vi "bats.parser.common.vi"(11 "BATS.Parser.State.Data in":T1={"BATS.Parser.States"=enum."Send.Command", "Saved.BATS.Parser.State"=enum."Reset", "Hdr Length (U16)"=0, "MessageLength (U8)"=0, "MessageType (U8)"=0, "Time (U32)"=0, "Total Counter (U16)"=0, "Message Counter (U8)"=0, "i"=0, "Number.of.Tickers"=0, "n"=0, "msg.counter"=0, "msg.length"=0, "buffer.start"=0, "buffer.length"=0, "buffer"=[0, 0, 0, 0, 0, 0, 0, 0, 0], "Debug"={"Write.to.Debug"=FALSE, "Data"=0}}) -> (1 "MessageType (U8)":u8, 2 "Message Counter (U8)":u8, 3 "BATS.Parser.State.Data out":T1={"BATS.Parser.States"=enum."Send.Command", "Saved.BATS.Parser.State"=enum."Reset", "Hdr Length (U16)"=0, "MessageLength (U8)"=0, "MessageType (U8)"=0, "Time (U32)"=0, "Total Counter (U16)"=0, "Message Counter (U8)"=0, "i"=0, "Number.of.Tickers"=0, "n"=0, "msg.counter"=0, "msg.length"=0, "buffer.start"=0, "buffer.length"=0, "buffer"=[0, 0, 0, 0, 0, 0, 0, 0, 0], "Debug"={"Write.to.Debug"=FALSE, "Data"=0}})   [LabVIEW 2022 SP3]
uses:
  bats.parser.state.command.ctl
  bats.parser.state.data.ctl
  debug/debug.type.ctl
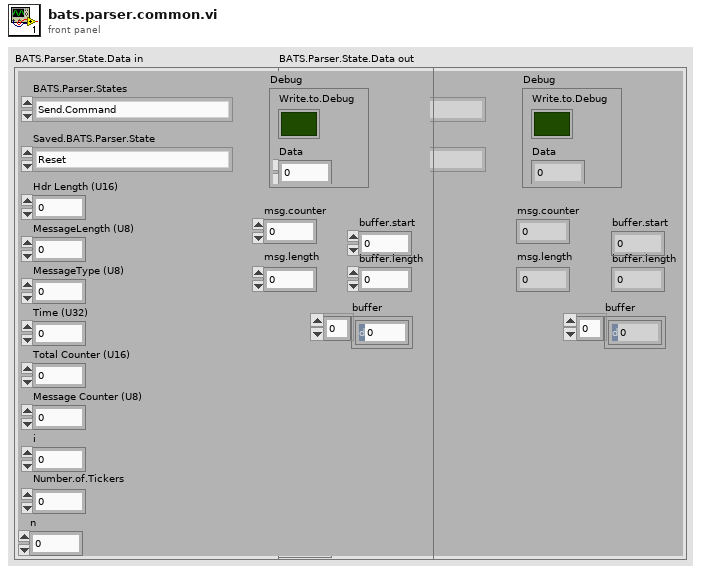
[diagram p1: front panel]
types:
  T1 = typedef "bats.parser.state.data.ctl" = cluster{"BATS.Parser.States":T2, "Saved.BATS.Parser.State":T2, "Hdr Length (U16)":u16, "MessageLength (U8)":u8, "MessageType (U8)":u8, "Time (U32)":u32, "Total Counter (U16)":u16, "Message Counter (U8)":u8, "i":u16, "Number.of.Tickers":u16, "n":u16, "msg.counter":u8, "msg.length":u8, "buffer.start":u8, "buffer.length":u8, "buffer":u64[], "Debug":T3}
  T2 = typedef "bats.parser.state.command.ctl" = enum16{"Reset", "Noop", "Read.Sequenced.Unit.Header", "Read.Msg", "Send.Command"}
  T3 = typedef "debug.type.ctl" = cluster{"Write.to.Debug":bool, "Data":u64}
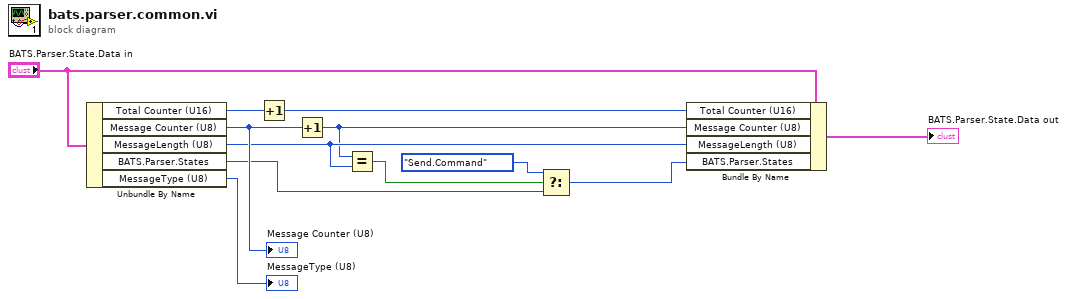
[diagram p0: block diagram]
diagram:
  n1 = Unbundle By Name("BATS.Parser.State.Data in") -> ("Total Counter (U16)"=w3:u16, "Message Counter (U8)"=w12:u8, "MessageLength (U8)"=w9:u8, "BATS.Parser.States"=w10:T2, "MessageType (U8)"=→"MessageType (U8)":u8)
  "Message Counter (U8)" <- w12
  n2 = Increment(x=w3) -> (x+1=w1:u16)
  n3 = Increment(x=w12) -> (x+1=w4:u8)
  n4 = Equal?(x=w4, y=w9) -> (x = y?=w5:bool)
  n5 = Select(t=bats.parser.state.command."Send.Command" ("BATS.Parser.States"), s=w5, f=w10) -> (s? t:f=w2:T2)
  n6 = Bundle By Name(cluster="BATS.Parser.State.Data in", "Total Counter (U16)"=w1, "Message Counter (U8)"=w4, "MessageLength (U8)"=w9, "BATS.Parser.States"=w2) -> (→"BATS.Parser.State.Data out":T1)
